vi "niFpgaPID_PICore.vi"(0 "setpoint":sgl, 1 "reset? (F)":bool, 3 "channel (0)":u8, 5 "process variable":sgl, 7 "manual control":T3, 12 "gains":T2 {"proportional gain" step=0.125}, 13 "output range":T4={"output high (Inf)"=inf, "output low (-Inf)"=-inf}, 14 "proportional weighting (1)":sgl=1.0 min=0 max=1) -> (4 "output":sgl, 6 "error":sgl, 8 "actions":T1)   [LabVIEW 2017]
uses:
  <vilib>/rvi/Analysis/control/PID/Typedef/niFpgaPID_OutputRange.ctl
  <vilib>/rvi/Analysis/control/PID/Typedef/niFpgaPID_ManualControl.ctl
  <vilib>/rvi/Analysis/control/PID/Typedef/niFpgaPID_PIGains.ctl
  <vilib>/rvi/Analysis/control/PID/Typedef/niFpgaPID_PIActions.ctl
  <vilib>/rvi/Analysis/control/PID/Typedef/niFpgaPID_PIErrors.ctl
  <vilib>/rvi/Analysis/control/PID/Typedef/niFpgaPID_PIParameters.ctl
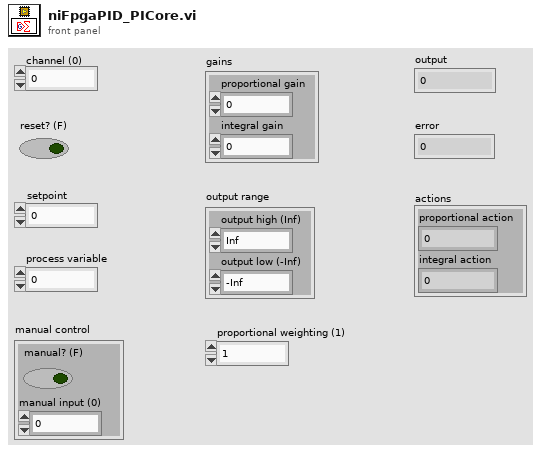
[diagram p1: front panel]
types:
  T1 = typedef "niFpgaPID_PIActions.ctl" = cluster{"proportional action":sgl, "integral action":sgl}
  T2 = typedef "niFpgaPID_PIGains.ctl" = cluster{"proportional gain":sgl, "integral gain":sgl}
  T3 = typedef "niFpgaPID_ManualControl.ctl" = cluster{"manual? (F)":bool, "manual input (0)":sgl}
  T4 = typedef "niFpgaPID_OutputRange.ctl" = cluster{"output high (Inf)":sgl, "output low (-Inf)":sgl}
  T5 = typedef "niFpgaPID_PIParameters.ctl" = cluster{"Kp":sgl, "Ki":sgl, "manual?":bool, "beta":sgl}
  T6 = typedef "niFpgaPID_PIErrors.ctl" = cluster{"error":sgl, "error with beta":sgl}
  T7 = typedef "niFpgaPID_PIState.ctl" = cluster{"uI(k-1)":sgl, "e(k-1)":sgl, "output (k-1)":sgl}
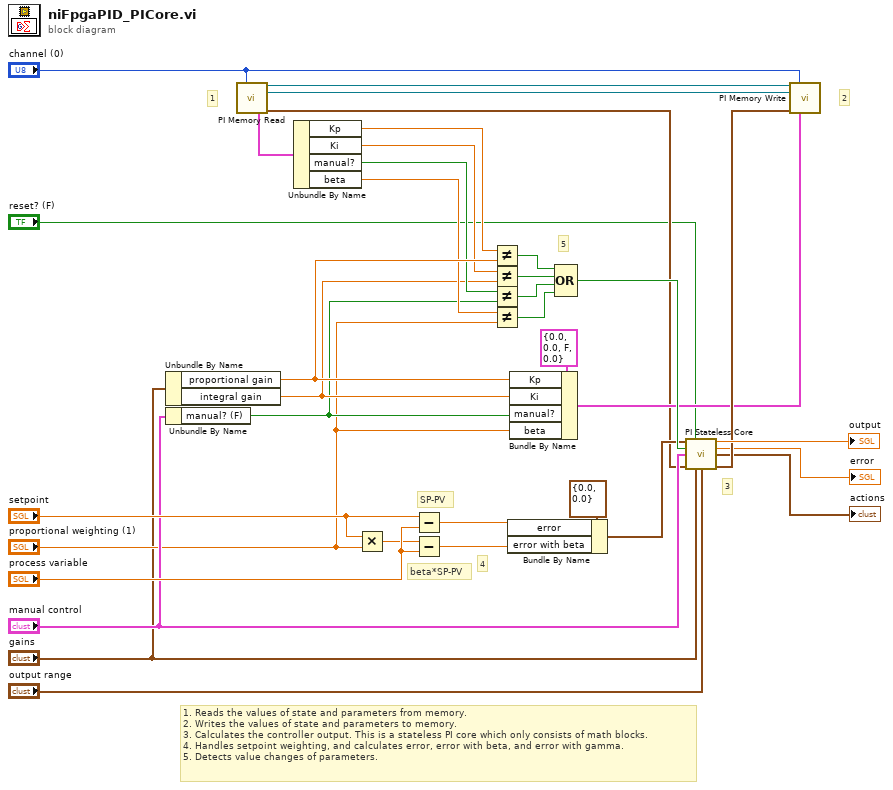
[diagram p0: block diagram]
diagram:
  # "1. Reads the values of state and parameters from memory.\n2. Writes the values of state and parameters to memory.\n3. Calculates the controller output. This is a stateless PI core which only consists of math blocks.\n4. Handles setpoint weighting, and calculates error, error with beta, and error with gamma.\n5. Detects value changes of parameters."
  # "SP-PV"
  # "beta*SP-PV"
  # "5"
  # "4"
  # "3"
  # "2"
  # "1"
  n1 = Unbundle By Name("gains") -> ("proportional gain"=w32:sgl, "integral gain"=w26:sgl)
  n2 = Unbundle By Name("manual control") -> ("manual? (F)"=w13:bool)
  n3 = call "PI Memory Read"("channel (0)"="channel (0)") -> ("data memory out"=w7:refnum<k21>, "manual memory out"=w6:refnum<k21>, "parameters out"=w20:T5, "state out"=w8:T7)  [unwired: 11 in]
  n4 = Unbundle By Name(w20) -> ("Kp"=w30:sgl, "Ki"=w29:sgl, "manual?"=w28:bool, "beta"=w27:sgl)
  n5 = Multiply(x="setpoint", y="proportional weighting (1)") -> (x*y=w2:sgl)
  n6 = Subtract(x="setpoint", y="process variable") -> (x-y=w4:sgl)
  n7 = Subtract(x=w2, y="process variable") -> (x-y=w18:sgl)
  n8 = Not Equal?(x=w30, y=w32) -> (x != y?=w25:bool)
  n9 = Not Equal?(x=w29, y=w26) -> (x != y?=w24:bool)
  n10 = Not Equal?(x=w28, y=w13) -> (x != y?=w11:bool)
  n11 = Not Equal?(x=w27, y="proportional weighting (1)") -> (x != y?=w10:bool)
  n12 = Bundle By Name(cluster=T6 {"error"=0.0, "error with beta"=0.0} ("errors"), "error"=w4, "error with beta"=w18) -> (w17:T6)
  n13 = Bundle By Name(cluster=T5 {"Kp"=0.0, "Ki"=0.0, "manual?"=FALSE, "beta"=0.0} ("parameters"), "Kp"=w32, "Ki"=w26, "manual?"=w13, "beta"="proportional weighting (1)") -> (w19:T5)
  n14 = Compound Arithmetic op=OR(w25, w24, w11, w10) -> (w33:bool)
  n15 = call "PI Stateless Core"("errors"=w17, "reset? (F)"="reset? (F)", "enable bumpless transfer? (F)"=w33, "manual control"="manual control", "state in"=w8, "gains"="gains", "output range"="output range") -> ("output"=→"output":sgl, "error"=→"error":sgl, "actions"=→"actions":T1, "state out"=w31:T7)  [unwired: 5 in]
  n16 = call "PI Memory Write"("data memory in"=w7, "channel (0)"="channel (0)", "manual memory in"=w6, "state in"=w31, "parameters in"=w19) -> ()  [unwired: 11 in]
